vi "static daq cluster generator.vi"(1 "time entry":dbl format="%.2f", 2 "voltage entry":dbl format="%.2f", 3 "DAQ channel\n number":u8, 4 "Input Array":T1(array[cluster]) {"Voltages" format="%.2f"; "Times" format="%.2f"}) -> (0 "Output Array":T1(array[cluster]) {"Voltages" format="%.2f"; "Times" format="%.2f"})   [LabVIEW 2015]
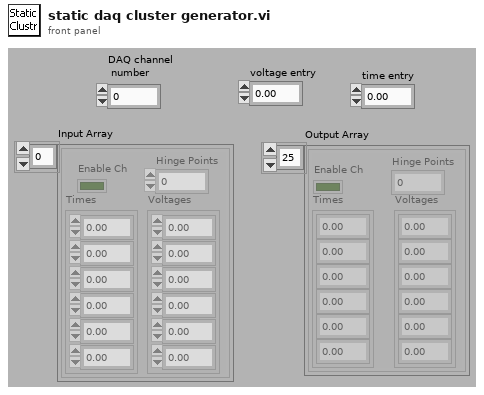
[diagram p1: front panel]
types:
  T1 = cluster{"Times":dbl[], "Voltages":dbl[], "Enable Ch":bool, "Hinge Points":u8}[]
  T2 = cluster{"Times":dbl[], "Voltages":dbl[], "Enable Ch":bool, "Hinge Points":u8}
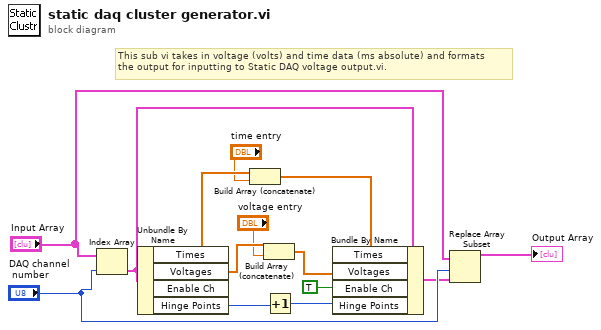
[diagram p0: block diagram]
diagram:
  # "This sub vi takes in voltage (volts) and time data (ms absolute) and formats\nthe output for inputting to Static DAQ voltage output.vi."
  n1 = Index Array(array="Input Array", index="DAQ channel\n number") -> (element=w14:T2)
  n2 = Unbundle By Name(w14) -> ("Times"=w12:dbl[], "Voltages"=w9:dbl[], "Hinge Points"=w3:u8)  [unwired: 1 out]
  n3 = Build Array (concatenate)(w12, "time entry") -> (w10:dbl[])
  n4 = Build Array (concatenate)(w9, "voltage entry") -> (w7:dbl[])
  n5 = Increment(x=w3) -> (x+1=w2:u8)
  n6 = Bundle By Name(cluster=w14, "Times"=w10, "Voltages"=w7, "Enable Ch"=TRUE, "Hinge Points"=w2) -> (w6:T2)
  n7 = Replace Array Subset(array="Input Array", new element=w6, index="DAQ channel\n number") -> (→"Output Array":T1)
